vi "Laser Current.vi"() -> ()   [LabVIEW 2010]
panel:
  out "Current (mA) 2":dbl
  in  "Current (mA)":dbl(slide) scale=0.0..75.0
  out "Dummy":string
  in  "Laser GPIB":u8=10 max=100
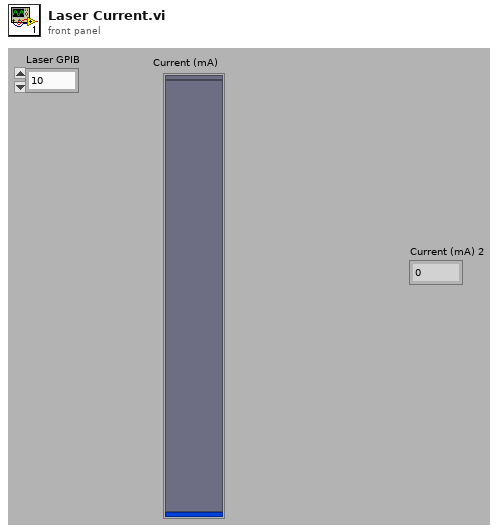
[diagram p1: front panel]
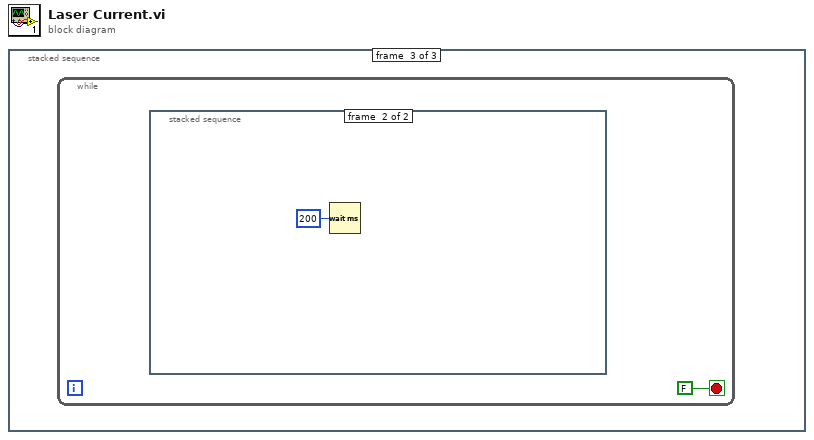
[diagram p0: block diagram]
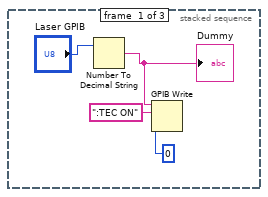
[diagram p2: hidden frame]
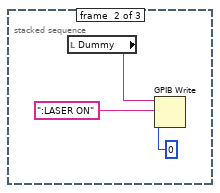
[diagram p3: hidden frame]
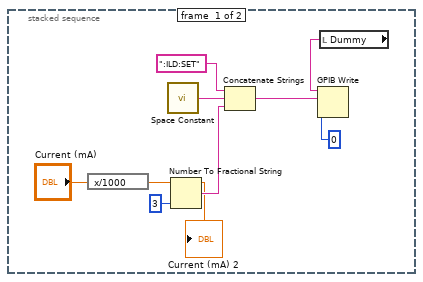
[diagram p4: hidden frame]
diagram:
  n1 = stacked-sequence {
    frame #0 {
      n2 = Number To Decimal String(number="Laser GPIB") -> (decimal integer string=w2:string)  [unwired: 1 in]
      "Dummy" <- w2
      n3 = GPIB Write(0:w2, 1:":TEC ON" ("data"), 2:i16 0 ("mode (0)")) -> ()  [unwired: 2 in, 2 out]
    }
    frame #1 {
      n4 = local read "Dummy"() -> (w6:string)
      n5 = GPIB Write(0:w6, 1:":LASER ON" ("data"), 2:i16 0 ("mode (0)")) -> ()  [unwired: 2 in, 2 out]
    }
    frame #2 {
      n6 = while {
        stop <- FALSE stop-if-true
        n7 = stacked-sequence {
          frame #0 {
            n8 = expression code="x/1000"("Current (mA)") -> (w13:dbl)
            n9 = call <vilib>:"Space Constant.vi"() -> ("String"=w11:string)
            n10 = Number To Fractional String(number=w13, precision (6)=i16 3) -> (F-format string=w16:string)  [unwired: 2 in]
            n11 = Concatenate Strings(":ILD:SET", w11, w16) -> (w12:string)
            n12 = local read "Dummy"() -> (w17:string)
            n13 = GPIB Write(0:w17, 1:w12, 2:i16 0 ("mode (0)")) -> ()  [unwired: 2 in, 2 out]
            "Current (mA) 2" <- "Current (mA)"
          }
          frame #1 {
            n14 = Wait (ms)(milliseconds to wait=u32 200) -> ()  [unwired: 1 out]
          }
        }
      }
    }
  }
